vi "专用-从新定时配置生成导出条件.vi"(11 "定时配置":T1={"定时模式"=enum."绝对时间", "单位"=enum."年", "间隔"=1, "目标时刻"=timestamp(0 s since 1904-01-01)} {"间隔" min=1}) -> (1 "时间上限(不含)":timestamp, 3 "时间下限(包含)":timestamp)   [LabVIEW 2017]
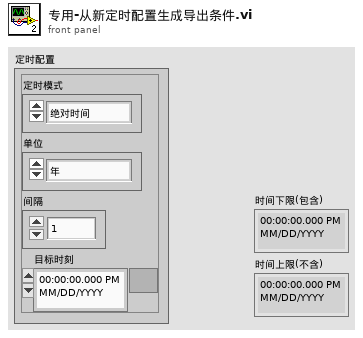
[diagram p1: front panel]
types:
  T1 = typedef "簇-定时配置.ctl" = cluster{"定时模式":enum16{"绝对时间", "相对时间"}, "单位":enum16{"年", "月", "日", "时", "分"}, "间隔":u8, "目标时刻":timestamp}
  T2 = typedef "LVDateTimeRec.ctl" = cluster{"秒数的小数部分":dbl, "秒":i32, "分":i32, "时":i32, "日":i32, "月":i32, "年":i32, "天数（周）":i32, "天数（年）":i32, "DST":i32}
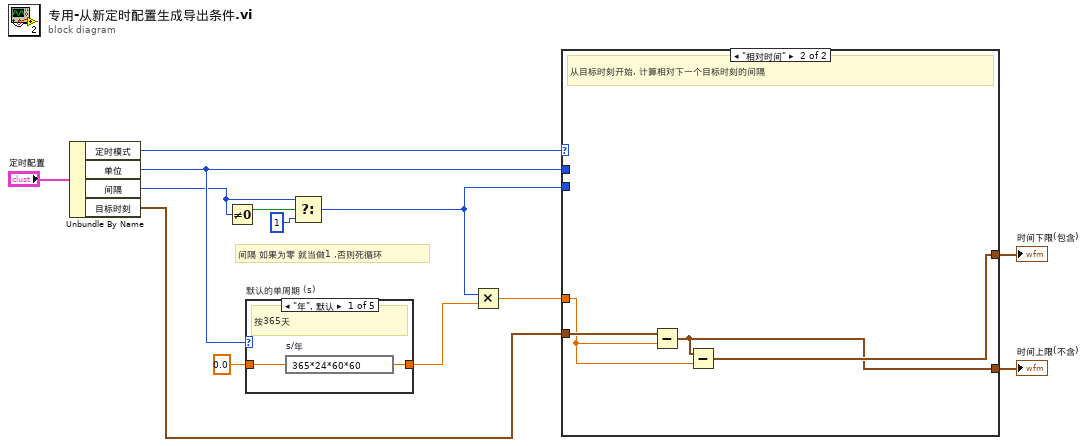
[diagram p0: block diagram]
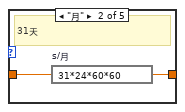
[diagram p2: hidden frame]
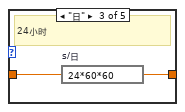
[diagram p3: hidden frame]
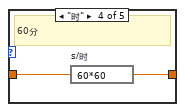
[diagram p4: hidden frame]
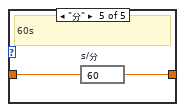
[diagram p5: hidden frame]
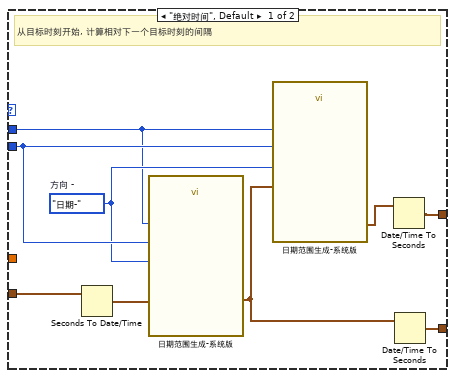
[diagram p6: hidden frame]
diagram:
  # "间隔 如果为零 就当做1 ,否则死循环"
  n1 = Unbundle By Name("定时配置") -> ("定时模式"=w6:enum16{"绝对时间", "相对时间"}, "单位"=w5:enum16{"年", "月", "日", "时", "分"}, "间隔"=w4:u8, "目标时刻"=w3:timestamp)
  n2 = Not Equal To 0?(x=w4) -> (x != 0?=w9:bool)
  n3 = case "默认的单周期 (s)" shown="\"年\", 默认" w5 {
    tunnel: [w15 w17 w19 w21 w23] -> w7
    tunnel: 0.0 -> [w14 w16 w18 w20 w22]
    frame "年", Default {
      # "按365天"
      n4 = expression code="365*24*60*60" "s/年"(w14) -> (w15:dbl)
    }
    frame "月" {
      # "31天"
      n5 = expression code="31*24*60*60" "s/月"(w16) -> (w17:dbl)
    }
    frame "日" {
      # "24小时"
      n6 = expression code="24*60*60" "s/日"(w18) -> (w19:dbl)
    }
    frame "时" {
      # "60分"
      n7 = expression code="60*60" "s/时"(w20) -> (w21:dbl)
    }
    frame "分" {
      # "60s"
      n8 = expression code="60" "s/分"(w22) -> (w23:dbl)
    }
  }
  n9 = Select(t=w4, s=w9, f=u8 1 ("间隔")) -> (s? t:f=w10:u8)
  n10 = Multiply(x=w10, y=w7) -> (x*y=w8:dbl)
  n11 = case shown="\"相对时间\"" w6 {
    tunnel: w5 -> [w26 _]
    tunnel: w10 -> [w28 _]
    tunnel: w3 -> [w31 w36]
    tunnel: w8 -> [_ w35]
    tunnel: [w30 w34] -> w1
    tunnel: [w29 w33] -> w2
    frame "绝对时间", Default {
      w27 = enum16{"当前", "日期+", "日期-"}."日期-"  # 方向 -
      # "从目标时刻开始, 计算相对下一个目标时刻的间隔"
      n12 = Seconds To Date/Time(time stamp (now)=w31) -> (date time rec=w32:T2)  [unwired: 1 in]
      n13 = call "日期范围生成-系统版.vi"("单位"=w26, "方向"=w27, "变化量(1)"=w28, "日期时间记录"=w32) -> ("下限"=w25:T2)  [unwired: 6 in, 1 out]
      n14 = call "日期范围生成-系统版.vi"("单位"=w26, "方向"=w27, "变化量(1)"=w28, "日期时间记录"=w25) -> ("下限"=w24:T2)  [unwired: 6 in, 1 out]
      n15 = Date/Time To Seconds(2:w24) -> (0:w30:timestamp)  [unwired: 1 in]
      n16 = Date/Time To Seconds(2:w25) -> (0:w29:timestamp)  [unwired: 1 in]
    }
    frame "相对时间" {
      # "从目标时刻开始, 计算相对下一个目标时刻的间隔"
      n17 = Subtract(x=w36, y=w35) -> (x-y=w33:timestamp)
      n18 = Subtract(x=w33, y=w35) -> (x-y=w34:timestamp)
    }
  }
  "时间下限(包含)" <- w1
  "时间上限(不含)" <- w2
